vi "Rot2Eul.vi"(1 "R":T1 caption="Real Matrix") -> (0 "E":dbl[](array[numeric]))   [LabVIEW 2018]
uses:
  <vilib>/Analysis/Matrix/Datatypes/RealMatrix.ctl
  <vilib>/Analysis/Matrix/Numeric/Conversions/Matrix To Array - RM.vi
  <vilib>/imath/engines/lvmath2/RunTimeEngine/IndexRead/NIMS M(S,S).vi
  <instcachedir>/0/NIMS M(S,S)_AC51E74150A542F7991B9634C66F3096.lvgen/NIMS M(S,S)_AC51E74150A542F7991B9634C66F3096_000.vi
  <vilib>/imath/engines/lvmath2/RunTimeEngine/BuiltInFunctions/abs/NIMS_abs(signed).vi
  <instcachedir>/0/NIMS_abs(signed)_C4FCB8E6058B49B797C7C8D53CA5F6EC.lvgen/NIMS_abs(signed)_C4FCB8E6058B49B797C7C8D53CA5F6EC_000.vi
  <vilib>/imathl/engines/lvmath/Functions/Error Handling/Create Error.vi
  <vilib>/imath/engines/lvmath2/RunTimeEngine/BuiltInFunctions/atan2/NIMS_atan2.vi
  <instcachedir>/0/NIMS_atan2_A91AA4A7D42247EDBE8F76DB99AF04A4.lvgen/NIMS_atan2_A91AA4A7D42247EDBE8F76DB99AF04A4_002.vi
  <vilib>/imath/engines/lvmath2/RunTimeEngine/ErrorHandling/NIMS_Create Error From Enums.vi
  <vilib>/imath/engines/lvmath2/RunTimeEngine/BuiltInFunctions/cos/NIMS_cos(C).vi
  <instcachedir>/0/NIMS_cos(C)_96B8A70E6B8E4D29AD8526A89C8CF3DF.lvgen/NIMS_cos(C)_96B8A70E6B8E4D29AD8526A89C8CF3DF_001.vi
  <instcachedir>/0/NIMS_atan2_A91AA4A7D42247EDBE8F76DB99AF04A4.lvgen/NIMS_atan2_A91AA4A7D42247EDBE8F76DB99AF04A4_001.vi
  <vilib>/imath/engines/lvmath2/RunTimeEngine/NodeEndStatement/NIMS_NodeEndStatement_Output.vi
  <instcachedir>/0/NIMS_NodeEndStatement_Output_53EC0D466D134D7ABD903AC30B43404B.lvgen/NIMS_NodeEndStatement_Output_53EC0D466D134D7ABD903AC30B43404B_005.vi
  <vilib>/imath/engines/lvmath2/RunTimeEngine/ErrorHandling/NIMS_Finalize Error.vi
  <vilib>/Analysis/Matrix/NI_Matrix.lvlib
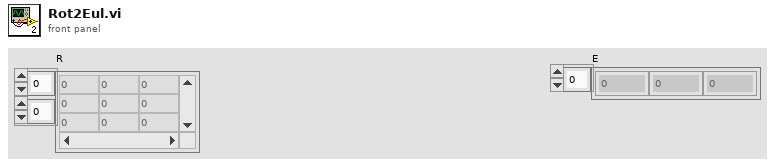
[diagram p1: front panel]
types:
  T1 = typedef "NI_Matrix.lvlib/RealMatrix.ctl" = dbl[][]
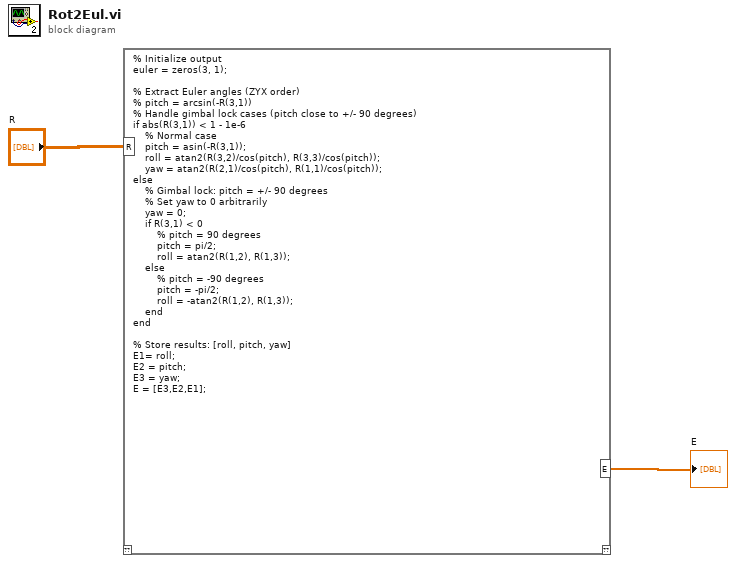
[diagram p0: block diagram]
diagram:
  n1 = mathscript code="% Initialize output\neuler = zeros(3, 1);\n\n% Extract Euler angles (ZYX order)\n% pitch = arcsin(-R(3,1))\n% Handle gimbal lock cases (pitch close to +/- 90 degrees)\nif abs(R(3,1)) < 1 - 1e-6\n    % Normal case\n    pitch = asin(-R(3,1));\n    roll = atan2(R(3,2)/cos(pitch), R(3,3)/cos(pitch));\n    yaw = atan2(R(2,1)/cos(pitch), R(1,1)/cos(pitch));\nelse\n    % Gimbal lock: pitch = +/- 90 degrees\n    % Set yaw to 0 arbitrarily\n    yaw = 0;\n    if R(3,1) < 0\n        % pitch = 90 degrees\n        pitch = pi/2;\n        roll = atan2(R(1,2), R(1,3));\n    else\n        % pitch = -90 degrees\n        pitch = -pi/2;\n        roll = -atan2(R(1,2), R(1,3));\n    end\nend\n\n% Store results: [roll, pitch, yaw]\nE1= roll;\nE2 = pitch;\nE3 = yaw;\nE = [E3,E2,E1];"("R"="R") -> ("E"=→"E":dbl[])  [unwired: 1 in, 1 out]
